vi "OAT Generate Time Indices.vi"(7 "reset? (True)":bool=TRUE, 9 "steps":cluster{"start":dbl, "end":dbl, "step":dbl} {"step" format="%.2f"; "end" format="%.2f"; "start" format="%.2f"}, 11 "duration":dbl format="%.2f") -> (0 "finished":bool, 1 "scale":cluster{"offset":dbl, "multiplier":dbl} {"multiplier" format="%.2f"; "offset" format="%.2f"}, 3 "time indices":dbl[](array[numeric]) format="%.2f", 5 "signal processed":dbl format="%.2f")   [LabVIEW 2017, in "SoundVib_Resampling.lvlib"]
uses:
  <vilib>/addons/Sound and Vibration/Order Analysis/Resample Order Tracking/SoundVib_Resampling.lvlib
  <vilib>/Analysis/NI_AALBase.lvlib
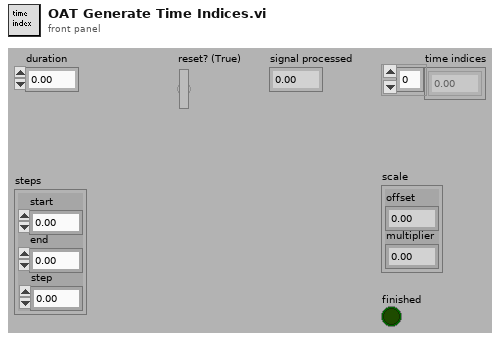
[diagram p1: front panel]
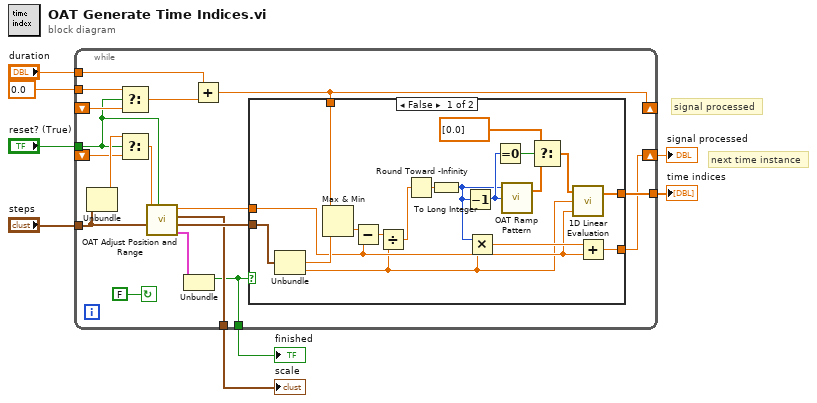
[diagram p0: block diagram]
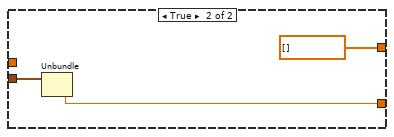
[diagram p2: hidden frame]
diagram:
  # "next time instance"
  # "signal processed"
  n1 = while {
    shift-right: [w11] -> w1
    shift-left: _ -> [w22]
    shift-right: [w16] -> _
    shift-left: _ -> [w25]
    tunnel: "steps" -> [w24]
    tunnel: "duration" -> [w21]
    tunnel: "reset? (True)" -> [w9]
    tunnel: 0.0 ("t") -> [w20]
    tunnel: [w17] -> w5
    tunnel: [w13] -> w4
    tunnel: [w15] -> w3
    stop <- FALSE continue-if-true
    n2 = Unbundle(w24) -> ("start"=w23:dbl)  [unwired: 2 out]
    n3 = Select(t=w20, s=w9, f=w25) -> (s? t:f=w14:dbl)
    n4 = Select(t=w23, s=w9, f=w22) -> (s? t:f=w12:dbl)
    n5 = call <vilib>:"OAT Adjust Position and Range.vi"("reset"=w9, "range in"=w24, "current position"=w12) -> ("flags"=w19:cluster{"finished":bool, "data missed":bool}, "range out"=w18:cluster{"start":dbl, "end":dbl, "step":dbl}, "scale"=w17:cluster{"offset":dbl, "multiplier":dbl}, "current position out"=w10:dbl)  [unwired: 5 in]
    n6 = Unbundle(w19) -> ("finished"=w13:bool)  [unwired: 1 out]
    n7 = Add(x=w21, y=w14) -> (x+y=w16:dbl)
    n8 = case shown="False" w13 {
      tunnel: w18 -> [w44 w46]
      tunnel: w16 -> [w40 _]
      tunnel: [w41 w45] -> w11
      tunnel: [w43 dbl[] [] ("Y[i]=X[i]*a+b")] -> w15
      tunnel: w10 -> [w32 _]
      frame False {
        n9 = Unbundle(w44) -> ("end"=w39:dbl, "step"=w30:dbl)  [unwired: 1 out]
        n10 = Max & Min(x=w40, y=w39) -> (min(x,y)=w38:dbl)  [unwired: 1 out]
        n11 = Subtract(x=w38, y=w32) -> (x-y=w31:dbl)
        n12 = Divide(x=w31, y=w30) -> (x/y=w29:dbl)
        n13 = Round Toward -Infinity(1:w29) -> (0:w27:dbl)
        n14 = To Long Integer(number=w27) -> (32bit integer=w28:i32)
        n15 = Decrement(x=w28) -> (x-1=w37:i32)
        n16 = Multiply(x=w28, y=w30) -> (x*y=w42:dbl)
        n17 = Equal To 0?(x=w37) -> (x = 0?=w36:bool)
        n18 = call <vilib>:"OAT Ramp Pattern.vi"("end"=w37, "samples"=w28) -> ("Ramp Pattern"=w34:dbl[])  [unwired: 1 in, 1 out]
        n19 = Select(t=dbl[] [0.0], s=w36, f=w34) -> (s? t:f=w35:dbl[])
        n20 = call <vilib>:"1D Linear Evaluation.vi"("offset"=w32, "scale"=w30, "X"=w35) -> ("Y[i]=X[i]*a+b"=w43:dbl[])  [unwired: 1 out]
        n21 = Add(x=w42, y=w32) -> (x+y=w41:dbl)
      }
      frame True {
        n22 = Unbundle(w46) -> ("start"=w45:dbl)  [unwired: 2 out]
      }
    }
  }
  "scale" <- w5
  "finished" <- w4
  "time indices" <- w3
  "signal processed" <- w1
